vi "PanelResizeControl.vi"(5 "TeleopDisplay":refnum<vi>, 6 "MainDashTab":refnum<vi>, 7 "TeleopSubPanel":refnum<vi>, 8 "stopButton":refnum<vi>, 9 "SubPanels":refnum<vi>[](array[refnum]), 10 "TopLevelVI":refnum<vi>, 11 "Plugin Info":T1) -> ()   [LabVIEW 2016]
uses:
  CorePluginInfo.ctl
  <vilib>/Utility/miscctls.llb/LVRectTypeDef.ctl
  <vilib>/Utility/miscctls.llb/LVPointTypeDef.ctl
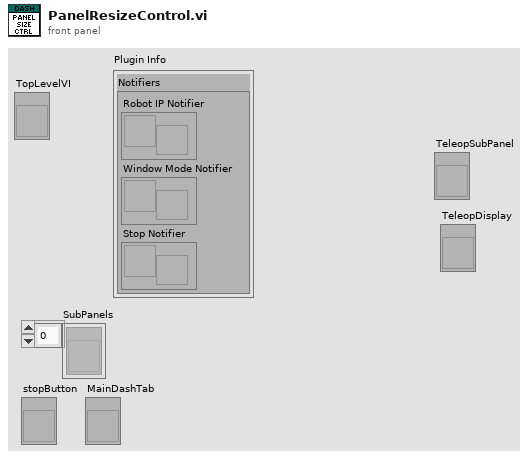
[diagram p1: front panel]
types:
  T1 = typedef "CorePluginInfo.ctl" = cluster{"Notifiers":cluster{"Robot IP Notifier":refnum<notifier>, "Window Mode Notifier":refnum<notifier>, "Stop Notifier":refnum<notifier>}}
  T2 = typedef "LVRectTypeDef.ctl" = cluster{"Left":i16, "Top":i16, "Right":i16, "Bottom":i16}
  T3 = typedef "LVPointTypeDef.ctl" = cluster{"Horizontal":i16, "Vertical":i16}
  T4 = enum16{"Always On", "Always Off", "Off While Running"}
  T5 = cluster{"TeleopSubPanel":refnum<vi>, "TeleopDisplay":refnum<vi>}
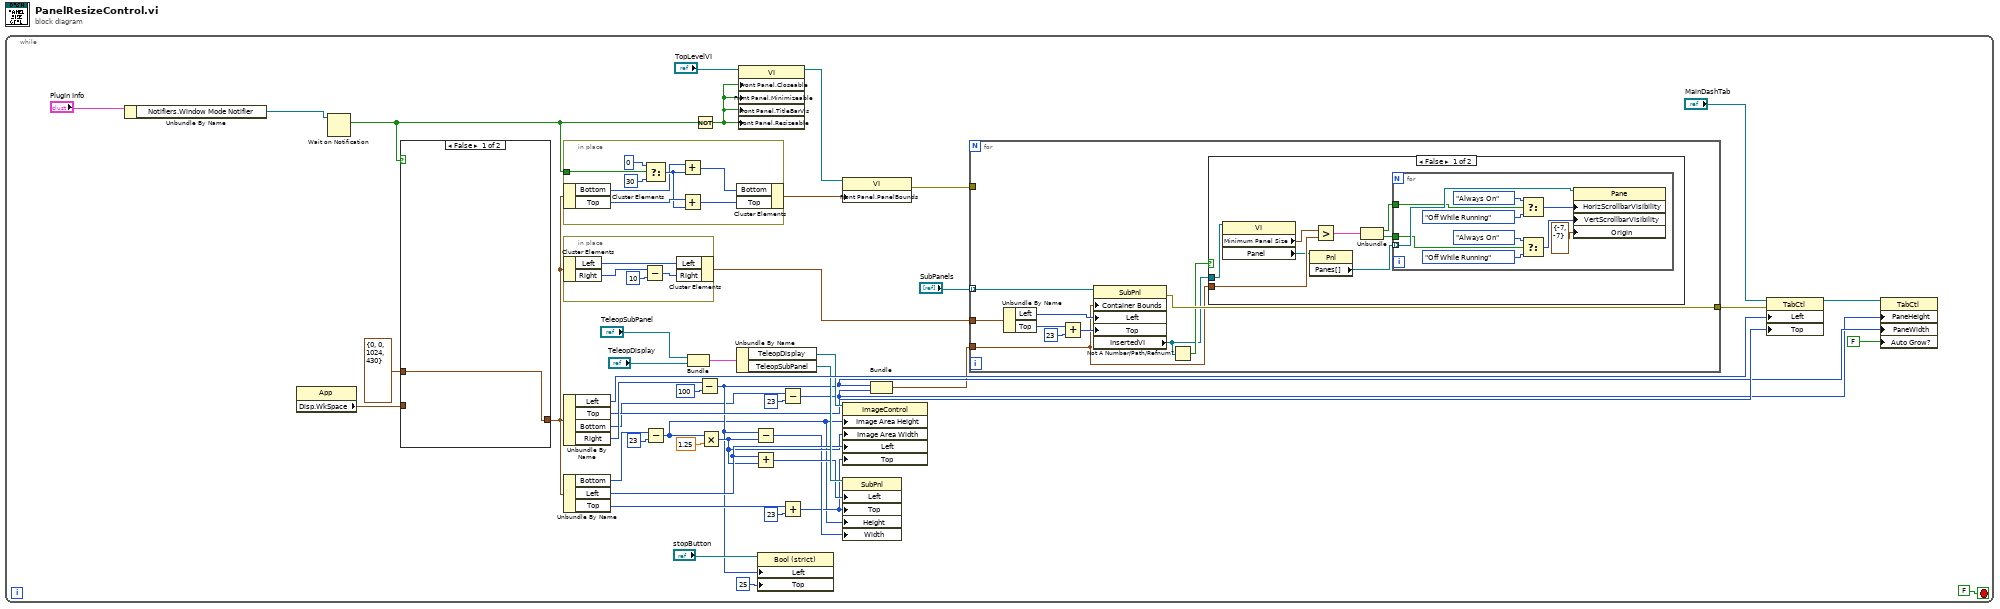
[diagram p0: block diagram]
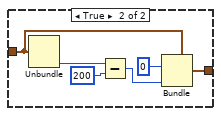
[diagram p3: hidden frame]
diagram:
  n1 = while {
    stop <- FALSE stop-if-true
    n2 = Unbundle By Name("Plugin Info") -> ("Notifiers.Window Mode Notifier"=w1:refnum<notifier>)
    n3 = property class="App"() -> ("Disp.WkSpace"=w45:T2)  [unwired: 2 in, 2 out]
    n4 = Wait on Notification(notifier=w1) -> (notification=w10:bool)  [unwired: 3 in, 3 out]
    n5 = case shown="False" w10 {
      tunnel: w45 -> [_ w88]
      tunnel: [w86 w89] -> w4
      tunnel: T2 {"Left"=0, "Top"=0, "Right"=1024, "Bottom"=430} ("Front Panel.PanelBounds") -> [w86 _]
      frame False {
      }
      frame True {
        n6 = Unbundle(w88) -> ("Bottom"=w92:i16)  [unwired: 3 out]
        n7 = Subtract(x=w92, y=200) -> (x-y=w90:i32)
        n8 = Bundle(cluster=w88, "Top"=i16 0, "Bottom"=w90) -> (w89:T2)  [unwired: 2 out]
      }
    }
    n9 = in-place {
      in-place-border: w10 -> [w81]
      n10 = in-place-cluster #1(w4) -> ("Bottom"=w78:i16, "Top"=w82:i16)
      n11 = Select(t=i16 0, s=w81, f=i16 30 ("Top")) -> (s? t:f=w80:i16)
      n12 = Add(x=w78, y=w80) -> (x+y=w79:i16)
      n13 = Add(x=w82, y=w80) -> (x+y=w83:i16)
      n14 = in-place-cluster #1("Bottom"=w79, "Top"=w83) -> (w11:T2)
    }
    n15 = in-place {
      n16 = in-place-cluster #2(w4) -> ("Left"=w74:i16, "Right"=w77:i16)
      n17 = Subtract(x=w77, y=i16 10) -> (x-y=w75:i16)
      n18 = in-place-cluster #2("Left"=w74, "Right"=w75) -> (w3:T2)
    }
    n19 = Unbundle By Name(w4) -> ("Left"=w43:i16, "Top"=w19:i16, "Bottom"=w17:i16, "Right"=w42:i16)
    n20 = Unbundle By Name(w4) -> ("Bottom"=w7:i16, "Left"=w35:i16, "Top"=w31:i16)
    n21 = Subtract(x=w7, y=i16 23) -> (x-y=w5:i16)
    n22 = Bundle("TeleopSubPanel"="TeleopSubPanel", "TeleopDisplay"="TeleopDisplay") -> (w38:T5)  [unwired: 1 in]
    n23 = Not(x=w10) -> (.not. x?=w12:bool)
    n24 = Subtract(x=w42, y=i16 100) -> (x-y=w18:i16)
    n25 = Multiply(x=w5, y=1.25) -> (x*y=w33:i32)
    n26 = Unbundle By Name(w38) -> ("TeleopDisplay"=w37:refnum<vi>, "TeleopSubPanel"=w36:refnum<vi>)
    n27 = property class="VI"(reference="TopLevelVI", "Front Panel.Closeable"=w12, "Front Panel.Minimizeable"=w12, "Front Panel.TitleBarVis"=w12, "Front Panel.Resizeable"=w12) -> (reference out=w44:refnum<vi>)  [unwired: 1 in, 1 out]
    n28 = Subtract(x=w18, y=w33) -> (x-y=w32:i32)
    n29 = Add(x=w35, y=w33) -> (x+y=w34:i32)
    n30 = property class="Bool (strict)"(reference="stopButton", "Left"=w18, "Top"=25 ("Position:Top")) -> ()  [unwired: 1 in, 2 out]
    n31 = Subtract(x=w17, y=i16 23) -> (x-y=w16:i16)
    n32 = Add(x=w31, y=i16 23) -> (x+y=w29:i16)
    n33 = property class="VI"(reference=w44, "Front Panel.PanelBounds"=w11) -> (error out=w14:errorcluster)  [unwired: 1 in, 1 out]
    n34 = property class="ImageControl"(reference=w37, "Image Area Height"=w5, "Image Area Width"=w33, "Left"=w35, "Top"=w29) -> ()  [unwired: 1 in, 2 out]
    n35 = property class="SubPnl"(reference=w36, "Left"=w34, "Top"=w29, "Height"=w5, "Width"=w32) -> ()  [unwired: 1 in, 2 out]
    n36 = Bundle(w18, w16) -> (w8:cluster{i16, i16})  [unwired: 1 in]
    n37 = for {
      tunnel: "SubPanels" -> [w55] mode=indexing
      tunnel: w3 -> [w54]
      tunnel: w8 -> [w48]
      tunnel: [w52] -> w20
      tunnel: w14 -> [_]
      n38 = Unbundle By Name(w54) -> ("Left"=w53:i16, "Top"=w51:i16)
      n39 = Add(x=w51, y=i16 23) -> (x+y=w50:i16)
      n40 = property class="SubPnl"(reference=w55, "Container Bounds"=w48, "Left"=w53, "Top"=w50) -> (error out=w52:errorcluster, "InsertedVI"=w46:refnum<vi>)  [unwired: 1 in, 1 out]
      n41 = Not A Number/Path/Refnum?(number/path/refnum=w46) -> (NaN/Path/Refnum?=w47:bool)
      n42 = case shown="False" w47 {
        tunnel: w46 -> [w63 _]
        tunnel: w48 -> [w61 _]
        frame False {
          n43 = property class="VI"(reference=w63) -> ("Minimum Panel Size"=w62:T3, "Panel"=w59:refnum<vi>)  [unwired: 1 in, 2 out]
          n44 = property class="Pnl"(reference=w59) -> ("Panes[]"=w58:refnum<vi>[])  [unwired: 1 in, 2 out]
          n45 = Greater?(x=w62, y=w61) -> (0:w60:cluster{bool, bool})
          n46 = Unbundle(w60) -> (w57:bool, w56:bool)
          n47 = for {
            tunnel: w58 -> [w73] mode=indexing
            tunnel: w57 -> [w69]
            tunnel: w56 -> [w66]
            n48 = Select(t=T4."Always On" ("Vertical Scrollbar Visibility"), s=w69, f=T4."Off While Running") -> (s? t:f=w71:T4)
            n49 = Select(t=T4."Always On" ("Vertical Scrollbar Visibility"), s=w66, f=T4."Off While Running") -> (s? t:f=w65:T4)
            n50 = property class="Pane"(reference=w73, "HorizScrollbarVisibility"=w71, "VertScrollbarVisibility"=w65, "Origin"=T3 {"Horizontal"=-7, "Vertical"=-7}) -> ()  [unwired: 1 in, 2 out]
          }
        }
        frame True {
        }
      }
    }
    n51 = property class="TabCtl"(reference="MainDashTab", error in=w20, "Left"=w43, "Top"=w19) -> (reference out=w9:refnum<vi>)  [unwired: 1 out]
    n52 = property class="TabCtl"(reference=w9, "PaneHeight"=w16, "PaneWidth"=w18, "Auto Grow?"=FALSE) -> ()  [unwired: 1 in, 2 out]
  }
